vi "LEP_RV_WriteObjectDataToXML.vi"(8 "error in":errorcluster, 10 "Object elements array":string[](array[string]), 11 "XMl file refnum":refnum<file>) -> (0 "error out":errorcluster)   [LabVIEW 2011]
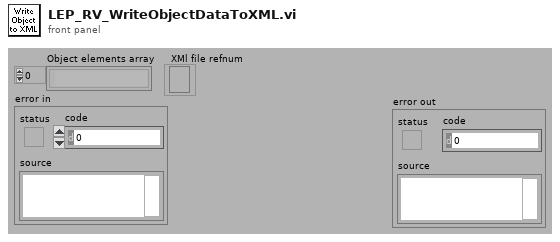
[diagram p1: front panel]
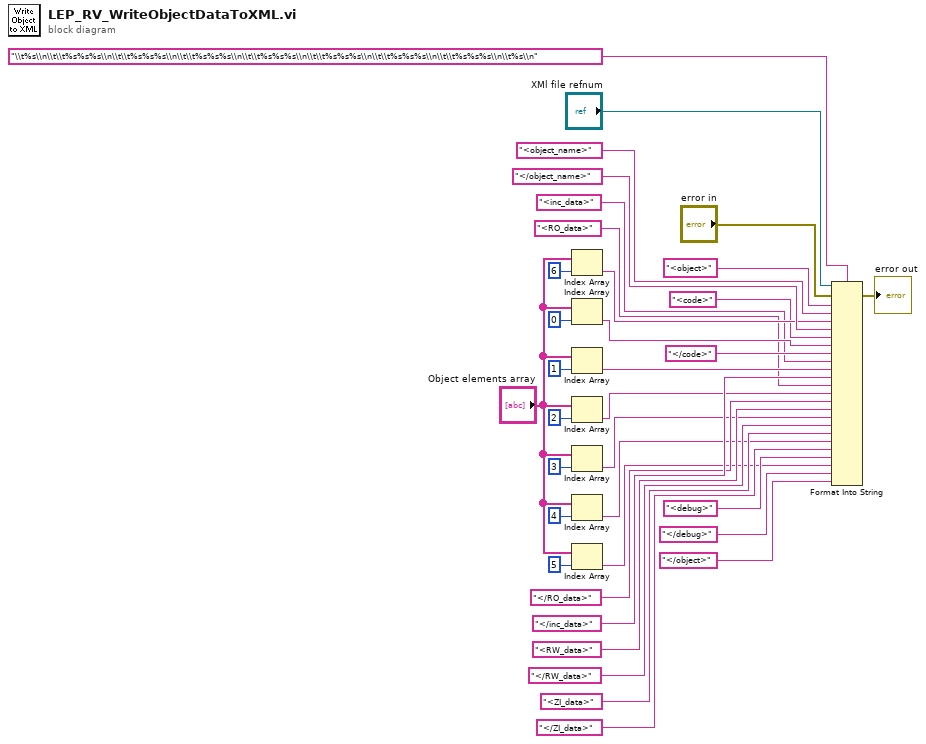
[diagram p0: block diagram]
diagram:
  n1 = Index Array(array="Object elements array", index=6) -> (element=w31:string)
  n2 = Index Array(array="Object elements array", index=0) -> (element=w23:string)
  n3 = Index Array(array="Object elements array", index=1) -> (element=w20:string)
  n4 = Index Array(array="Object elements array", index=2) -> (element=w16:string)
  n5 = Index Array(array="Object elements array", index=3) -> (element=w9:string)
  n6 = Index Array(array="Object elements array", index=4) -> (element=w6:string)
  n7 = Index Array(array="Object elements array", index=5) -> (element=w3:string)
  n8 = Format Into String(format string="\\t%s\\n\\t\\t%s%s%s\\n\\t\\t%s%s%s\\n\\t\\t%s%s%s\\n\\t\\t%s%s%s\\n\\t\\t%s%s%s\\n\\t\\t%s%s%s\\n\\t\\t%s%s%s\\n\\t%s\\n", initial string="XMl file refnum", error in="error in", "<object>" ("input 1"), "<object_name>" ("input 2"), w31, "</object_name>" ("input 3"), "<code>" ("input 5"), w23, "</code>" ("input 7"), "<inc_data>" ("input 5"), w20, "</inc_data>" ("input 7"), "<RO_data>" ("input 5"), w16, "</RO_data>" ("input 7"), "<RW_data>" ("input 5"), w9, "</RW_data>" ("input 7"), "<ZI_data>" ("input 5"), w6, "</ZI_data>" ("input 7"), "<debug>" ("input 5"), w3, "</debug>" ("input 7"), "</object>" ("input 1")) -> (error out=→"error out":errorcluster)  [unwired: 1 out]
